vi "Simple Reader.vi"(8 "error in (no error)":errorcluster, 11 "nanocal in":refnum<class "nanocal.lvclass">) -> (0 "error out":errorcluster, 2 "Signals":dbl[](array[numeric]), 3 "nanocal out":refnum<class "nanocal.lvclass">)   [LabVIEW 2019, in "nanocal.lvclass"]
uses:
  nanocal.lvclass
  data/github/NHMFL_Core/Libraries/Instruments/Instrument Driver/Instrument Driver.lvclass
  resonant_ultrasound_arxiv/maglab ultrasound -- arkady --arxiv/publisher action.ctl
  NHMFL_Core/Libraries/Instruments/Instrument Driver/Instrument Driver.lvclass/Instrument Driver.ctl
  NHMFL_Core/Libraries/Instruments/Instrument Driver/Write Channel names.vi
  NHMFL_Core/Libraries/Instruments/Instrument Driver/Write Channel units.vi
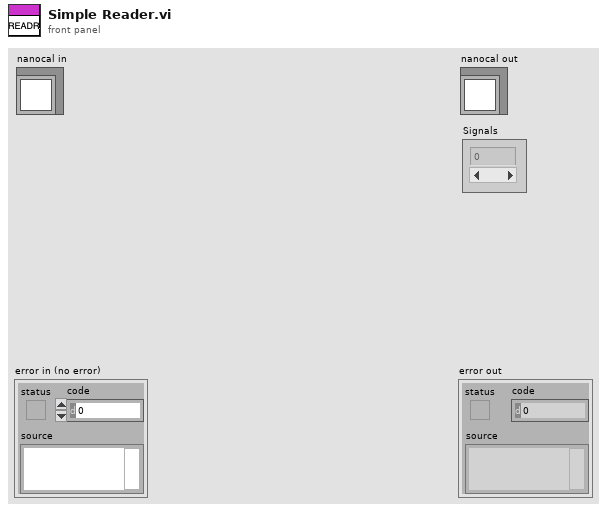
[diagram p1: front panel]
types:
  T1 = typedef "publisher action.ctl" = enum16{"set", "get", "init", "check"}
  T2 = typedef "icicle.ctl" = cluster{"name":string, "units":string, "data":dbl}
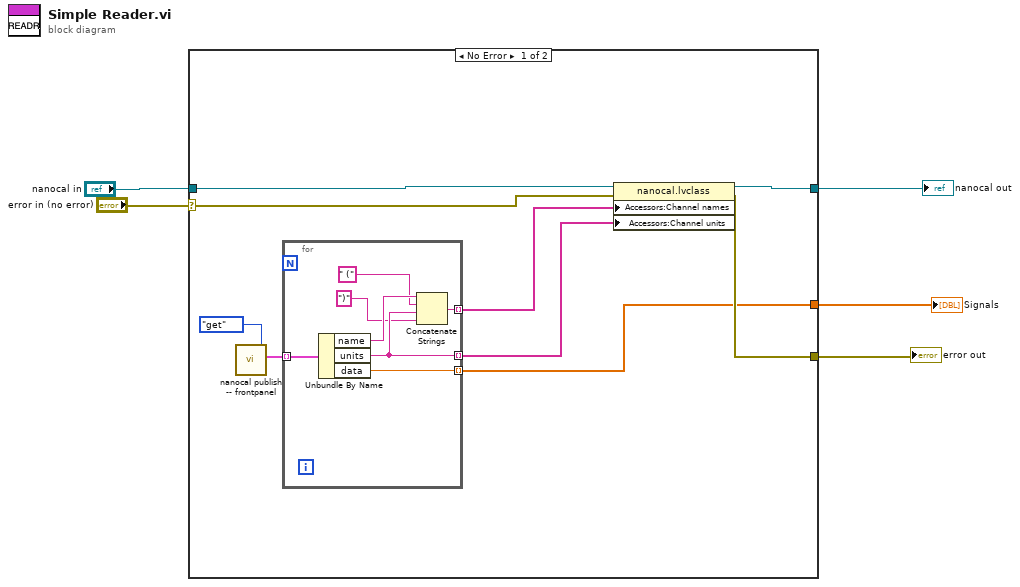
[diagram p0: block diagram]
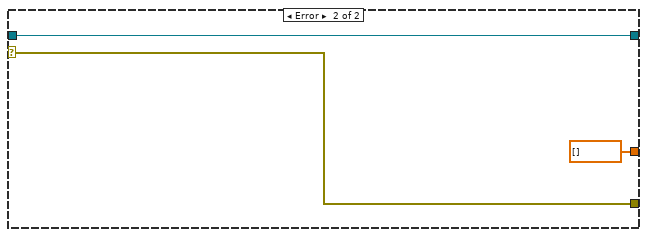
[diagram p2: hidden frame]
diagram:
  n1 = case shown="No Error" "error in (no error)" {
    selector: "error in (no error)" -> [w13 w24]
    tunnel: [w12 w24] -> w2
    tunnel: [w14 w23] -> w3
    tunnel: "nanocal in" -> [w10 w23]
    tunnel: [w6 dbl[] []] -> w1
    frame No Error {
      n2 = call "nanocal publish -- frontpanel.vi"("publisher action"=publisher_action."get") -> ("nanocal data array OUT"=w9:T2[])  [unwired: 10 in]
      n3 = for {
        tunnel: w9 -> [w21] mode=indexing
        tunnel: [w17] -> w8 mode=indexing
        tunnel: [w18] -> w7 mode=indexing
        tunnel: [w20] -> w6 mode=indexing
        n4 = Unbundle By Name(w21) -> ("name"=w19:string, "units"=w18:string, "data"=w20:dbl)
        n5 = Concatenate Strings(w19, " (", w18, ")") -> (w17:string)
      }
      n6 = property class="nanocal.lvclass"(reference=w10, error in=w13, "Accessors:Channel names"=w8, "Accessors:Channel units"=w7) -> (reference out=w14:refnum<class "nanocal.lvclass">, error out=w12:errorcluster)
    }
    frame Error {
    }
  }
  "error out" <- w2
  "nanocal out" <- w3
  "Signals" <- w1
